vi "PID Autotune X-Axis.vi"() -> ()   [LabVIEW 2017]
uses:
  <vilib>/addons/control/pid/autopid.llb/PID autotuning parameters (adv).ctl
  <vilib>/myRIO/Common/Instrument Driver Framework/myRIO v1.0/UART/vis/myRIO v1.0 Close UART.vi
  <vilib>/addons/control/pid/pid.llb/PID Control Input Filter (DBL).vi
  <vilib>/myRIO/Common/Instrument Driver Framework/Utilities/vis/FPGA Ref Manager.vi
  <vilib>/myRIO/Common/Instrument Driver Framework/myRIO v1.0/myRIO v1.0 Reset FPGA.vi
  <vilib>/myRIO/Common/Instrument Driver Framework/myRIO v1.0/IRQ/vis/myRIO v1.0 IRQ Info FGV.vi
  <vilib>/myRIO/Common/Instrument Driver Framework/myRIO v1.0/IRQ/vis/myRIO v1.0 Timer IRQ Info FGV.vi
  <vilib>/myRIO/Common/Instrument Driver Framework/myRIO v1.0/IRQ/vis/myRIO v1.0 ISR Agent.vi
  <vilib>/myRIO/Instrument Drivers/Utilities/Utilities.lvlib
  <vilib>/addons/control/pid/NI_PID_pid.lvlib
  <vilib>/addons/control/pid/NI_PID_autopid.lvlib
panel:
  in  "alpha":dbl=0.1 format="%.2f"
  in  "gamma":dbl format="%.2f"
  in  "autotuning parameters":T1={"technique"=2, "type of controller"=1, "control specification"=0, "amplitude"=1.0} {"amplitude" format="%.2f"; "control specification" items=["normal", "fast", "slow"]; "type of controller" items=["P", "PI", "PID"]; "technique" items=["Step Open Loop", "Step Closed Loop", "Relay", "PID Relay"]}
  in  "reinitialize? (F)":bool
  out "tuning completed?":bool
  in  "auto? (F)":bool
  out "tuned PID gains":T2={"proportional gain (Kc)"=1.0, "integral time (Ti, min)"=0.01, "derivative time (Td, min)"=0.0} {"derivative time (Td, min)" format="%#.6g"; "integral time (Ti, min)" format="%#.6g"; "proportional gain (Kc)" format="%#.6g"}
  in  "autotune? (F)":bool
  out "Sensor Output":cluster{dbl, "output":dbl}(graph)
  out "Motion Data":T3
  in  "FWD/RVS":bool
  out "Time (s)":dbl
  out "Output String":string
  out "PID Output":dbl(graph)
  out "SP & PV":T4(graph)
  in  "PID gains":T2={"proportional gain (Kc)"=1.0, "integral time (Ti, min)"=0.01, "derivative time (Td, min)"=0.0} {"derivative time (Td, min)" format="%.4f"; "integral time (Ti, min)" format="%.4f"; "proportional gain (Kc)" format="%.3f"}
  out "dt out (s)":dbl format="%.3f"
  in  "Frequency":dbl
  in  "Velocity Set Pt":dbl
  in  "stop":bool
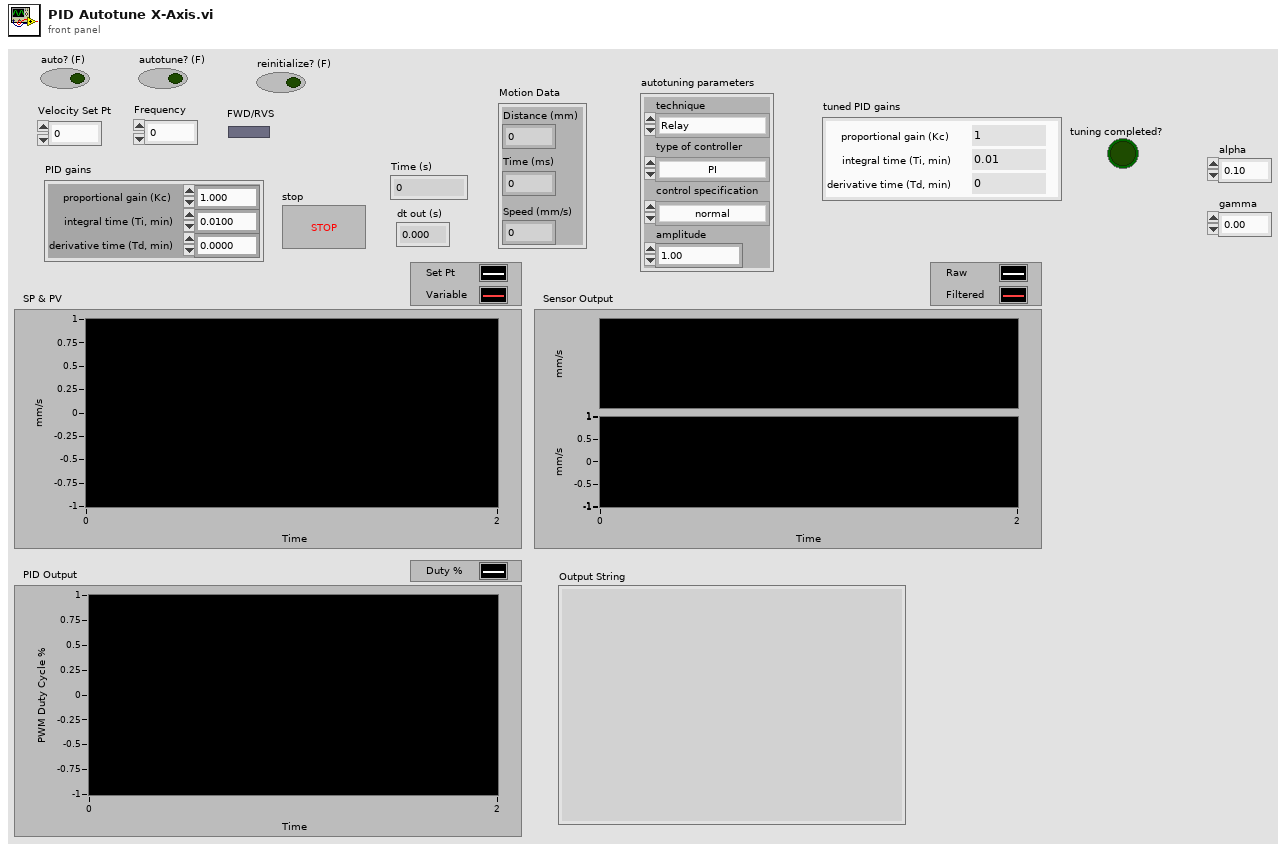
[diagram p1: front panel]
types:
  T1 = typedef "NI_PID_autopid.lvlib/PID autotuning parameters (adv).ctl" = cluster{"technique":u16, "type of controller":u16, "control specification":u16, "amplitude":dbl}
  T2 = cluster{"proportional gain (Kc)":dbl, "integral time (Ti, min)":dbl, "derivative time (Td, min)":dbl}
  T3 = cluster{"Distance (mm)":dbl, "Time (ms)":u32, "Speed (mm/s)":dbl}
  T4 = cluster{"Velocity Set Pt":dbl, "Velocity (mm/s)":dbl}
  T5 = cluster{"Velocity Set Pt":dbl, "Velocity (mm/s)":dbl}[]
  T6 = typedef "Encoder Cluster.ctl" = cluster{"Y-axis rev count":dbl, "Y-axis distance":dbl, "X-axis rev count":dbl, "X-axis distance":dbl, "Y-axis direction":T7, "X-axis direction":T7, "X-counter val":i32, "Y-counter val":i32}
  T7 = typedef "Encoder Count Direction Enum.ctl" = enum16{"Counting Up", "Counting Down"}
  T8 = cluster{dbl, "Velocity Set Pt":dbl, "output":dbl, "output":dbl, "proportional gain (Kc)":dbl, "integral time (Ti, min)":dbl, "derivative time (Td, min)":dbl}
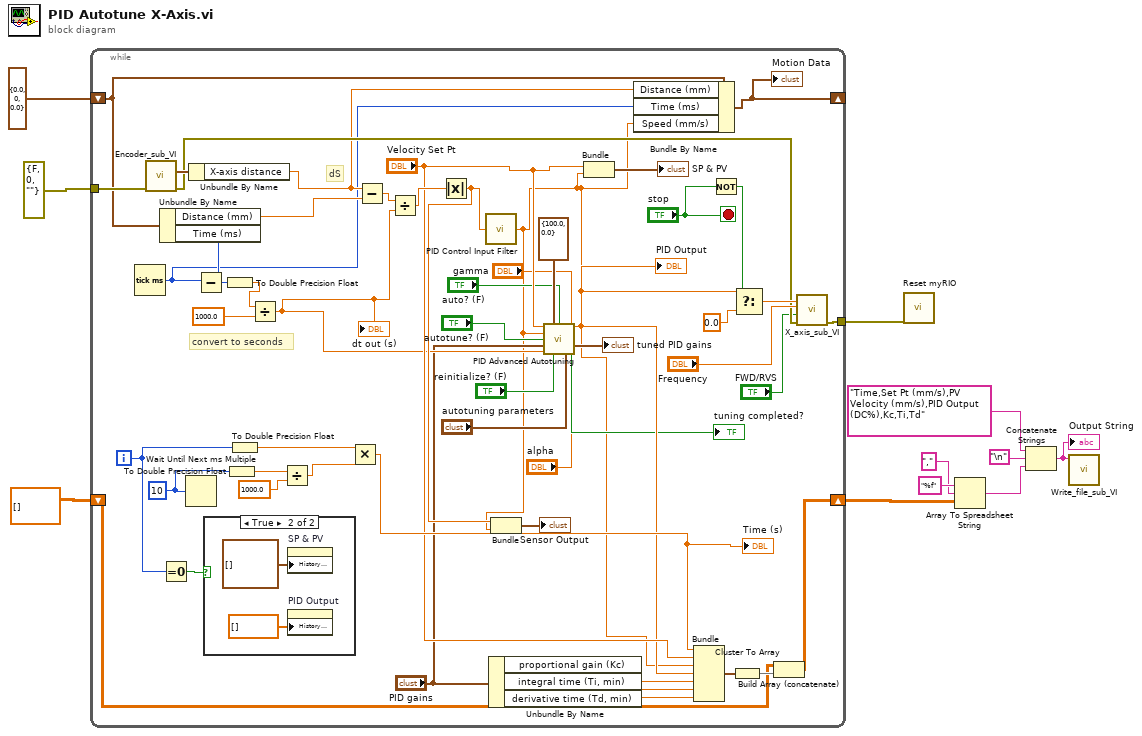
[diagram p0: block diagram]
diagram:
  n1 = while {
    shift-right: [w49] -> w4
    shift-left: dbl[][] [] ("element") -> [w50]
    tunnel: errorcluster {"status"=FALSE, "code"=0, "source"=""} ("error constant") -> [w48]
    tunnel: [w46] -> w2
    shift-right: [w28] -> _
    shift-left: T3 {"Distance (mm)"=0.0, "Time (ms)"=0, "Speed (mm/s)"=0.0} ("Motion Data") -> [w32]
    i -> [w34]
    stop <- "stop" stop-if-true
    w37 = u32 10 ("millisecond multiple")
    # "dS"
    # "convert to seconds"
    n2 = Tick Count (ms)() -> (millisecond timer value=w29:u32)
    n3 = call "Encoder_sub_VI.vi"("error in (no error)"=w48) -> ("error out"=w47:errorcluster, "Encoder Output"=w63:T6)  [unwired: 9 in]
    n4 = Unbundle By Name(w32) -> ("Distance (mm)"=w33:dbl, "Time (ms)"=w30:u32)
    n5 = Equal To 0?(x=w34) -> (x = 0?=w35:bool)
    n6 = Wait Until Next ms Multiple(millisecond multiple=w37) -> ()  [unwired: 1 out]
    n7 = Unbundle By Name(w63) -> ("X-axis distance"=w31:dbl)
    n8 = Subtract(x=w29, y=w30) -> (x-y=w54:u32)
    n9 = case shown="True" w35 {
      frame False {
      }
      frame True {
        n10 = property on="SP & PV" class="WFChart (strict)"("History Data"=T5 []) -> ()  [unwired: 2 in, 2 out]
        n11 = property on="PID Output" class="WFChart (strict)"("History Data"=dbl[] []) -> ()  [unwired: 2 in, 2 out]
      }
    }
    n12 = To Double Precision Float(number=w54) -> (double precision float=w53:dbl)
    n13 = To Double Precision Float(number=w37) -> (double precision float=w45:dbl)
    n14 = To Double Precision Float(number=w34) -> (double precision float=w38:dbl)
    n15 = Divide(x=w53, y=1000.0) -> (x/y=w23:dbl)
    "dt out (s)" <- w23
    n16 = Divide(x=w45, y=1000.0) -> (x/y=w40:dbl)
    n17 = Multiply(x=w38, y=w40) -> (x*y=w39:dbl)
    "Time (s)" <- w39
    n18 = Subtract(x=w31, y=w33) -> (x-y=w61:dbl)
    n19 = Divide(x=w61, y=w23) -> (x/y=w60:dbl)
    n20 = Absolute Value(x=w60) -> (abs(x)=w26:dbl)
    n21 = call-poly <vilib>:"PID Control Input Filter.vi"("input"=w26) -> ("output"=w12:dbl)  [unwired: 4 in]
    n22 = Unbundle By Name("PID gains") -> ("proportional gain (Kc)"=w43:dbl, "integral time (Ti, min)"=w42:dbl, "derivative time (Td, min)"=w41:dbl)
    n23 = Bundle(w26, "output"=w12) -> (→"Sensor Output":cluster{dbl, "output":dbl})  [unwired: 1 in]
    n24 = call <vilib>:"PID Advanced Autotuning.vi"("setpoint"="Velocity Set Pt", "output range"=cluster{"output high":dbl, "output low":dbl} {"output high"=100.0, "output low"=0.0}, "auto? (F)"="auto? (F)", "process variable"=w12, "gamma"="gamma", "autotune? (F)"="autotune? (F)", "alpha"="alpha", "PID gains"="PID gains", "dt (s)"=w23, "reinitialize? (F)"="reinitialize? (F)", "autotuning parameters"="autotuning parameters") -> ("output"=w20:dbl, "tuned PID gains"=→"tuned PID gains":T2, "tuning completed?"=→"tuning completed?":bool)  [unwired: 2 in]
    "PID Output" <- w20
    n25 = Bundle("Velocity Set Pt"="Velocity Set Pt", "output"=w12) -> (→"SP & PV":cluster{"Velocity Set Pt":dbl, "output":dbl})  [unwired: 1 in]
    n26 = Bundle By Name(cluster=w32, "Distance (mm)"=w31, "Time (ms)"=w29, "Speed (mm/s)"=w12) -> (w28:T3)
    "Motion Data" <- w28
    n27 = Bundle(w39, "Velocity Set Pt"="Velocity Set Pt", "output"=w12, "output"=w20, "proportional gain (Kc)"=w43, "integral time (Ti, min)"=w42, "derivative time (Td, min)"=w41) -> (w52:T8)  [unwired: 1 in]
    n28 = Not(x="stop") -> (.not. x?=w58:bool)
    n29 = Cluster To Array(cluster=w52) -> (array=w51:dbl[])
    n30 = Select(t=w20, s=w58, f=0.0) -> (s? t:f=w56:dbl)
    n31 = Build Array (concatenate)(w50, w51) -> (w49:dbl[][])
    n32 = call "X_axis_sub_VI.vi"("error in (no error)"=w47, "FWD/RVS"="FWD/RVS", "Frequency"="Frequency", "Duty Cycle %"=w56) -> ("error out"=w46:errorcluster)  [unwired: 7 in]
  }
  n33 = call <vilib>:"Reset myRIO.vi"("error in (no error)"=w2) -> ()  [unwired: 10 in, 1 out]
  n34 = Array To Spreadsheet String(delimiter (Tab)=",", array=w4, 3:"%f" ("format string")) -> (spreadsheet string=w10:string)
  n35 = Concatenate Strings("Time,Set Pt (mm/s),PV Velocity (mm/s),PID Output (DC%),Kc,Ti,Td", "\n", w10) -> (w9:string)
  "Output String" <- w9
  n36 = call "Write_file_sub_VI.vi"("Output String"=w9) -> ()  [unwired: 9 in, 2 out]
